vi "SubVI_Edge_Auto.vi"(8 "error in":errorcluster, 10 "Parameter_Edge":T3={"Parameter_Edge"={"ROI Descriptor"={"Global Rectangle"=[], "Contours"=[]}, "Edge Options"={"Edge Polarity"=0, "Kernel Size"=3, "Width"=3, "Minimum Edge Strength"=10.0, "Interpolation Type"=enum."Bilinear Fixed", "Data Processing Method"=enum."Average"}, "Scan Direction"=0, "Step Size"=5, "Auto"=FALSE}, "Group"="", "Color"=6618880, "Standard deviation"=0.0, "Pixel to Micrometer"=0.0, "Radius"=4} {"Parameter_Edge"."Edge Options"."Edge Polarity" items=["All Edges", "Rising Edges", "Falling Edges"]; "Parameter_Edge"."Edge Options"."Minimum Edge Strength" format="%.2f"; "Parameter_Edge"."Edge Options"."Width" step=2; "Parameter_Edge"."Edge Options"."Kernel Size" step=2; "Parameter_Edge"."Scan Direction" items=["Left To Right", "Right To Left", "Top To Bottom", "Bottom To Top"]; "Parameter_Edge"."ROI Descriptor"."Contours"."Type" items=["No Selection", "Point", "Line", "Rectangle", "Oval", "Polygon", "Free", "Annulus", "Unused2", "Unused3", "Broken Line", "Free Hand Line", "Rotated Rectangle"]}, 11 "Image in":T4) -> (0 "error out":errorcluster, 2 "Result_Edge":T5 {"MidPoint"."Y" format="%.2f"; "MidPoint"."X" format="%.2f"; "Line Segment"."Point 2"."Y" format="%.2f"; "Line Segment"."Point 2"."X" format="%.2f"; "Line Segment"."Point 1"."Y" format="%.2f"; "Line Segment"."Point 1"."X" format="%.2f"}, 3 "Image Out":T4)   [LabVIEW 2013]
uses:
  <vilib>/vision/Image Controls.llb/IMAQ Image.ctl
  <vilib>/vision/Measure.llb/Edge Options.ctl
  <vilib>/vision/Measure.llb/Edge Polarity.ctl
  <vilib>/vision/NI_Vision_Development_Module.lvlib
  <vilib>/Analysis/NI_AALBase.lvlib
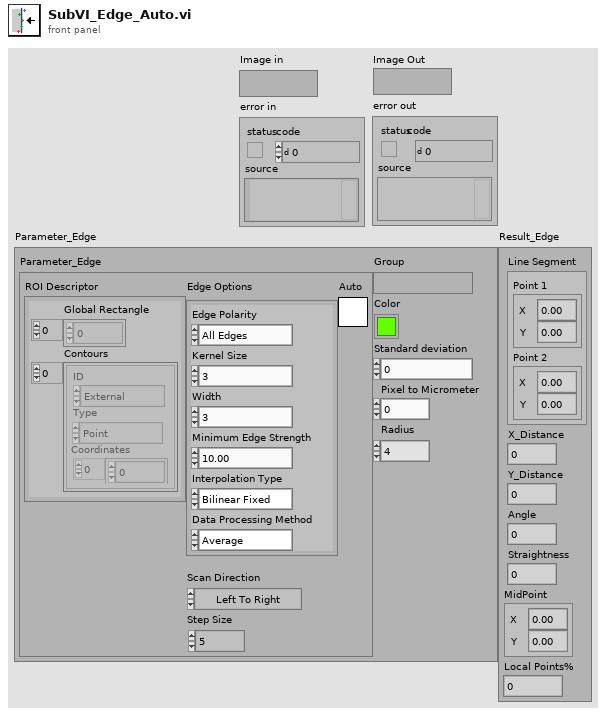
[diagram p1: front panel]
types:
  T1 = typedef "Edge Options.ctl" = cluster{"Edge Polarity":T2, "Kernel Size":u32, "Width":u32, "Minimum Edge Strength":sgl, "Interpolation Type":enum32{"Zero Order", "Bilinear", "Quadratic", "Cubic", "Bilinear Fixed"}, "Data Processing Method":enum32{"Average", "Median"}}
  T2 = typedef "Edge Polarity.ctl" = u32
  T3 = cluster{"Parameter_Edge":cluster{"ROI Descriptor":cluster{"Global Rectangle":i32[], "Contours":cluster{"ID":enum32{"External", "Internal"}, "Type":u32, "Coordinates":i32[]}[]}, "Edge Options":T1, "Scan Direction":u16, "Step Size":u32, "Auto":bool}, "Group":string, "Color":u32, "Standard deviation":dbl, "Pixel to Micrometer":dbl, "Radius":i32}
  T4 = typedef "IMAQ Image.ctl" = refnum<image>
  T5 = cluster{"Line Segment":cluster{"Point 1":cluster{"X":sgl, "Y":sgl}, "Point 2":cluster{"X":sgl, "Y":sgl}}, "X_Distance":dbl, "Y_Distance":dbl, "Angle":dbl, "Straightness":dbl, "MidPoint":cluster{"X":sgl, "Y":sgl}, "Local Points%":dbl}
  T6 = cluster{"ROI Descriptor":cluster{"Global Rectangle":i32[], "Contours":cluster{"ID":enum32{"External", "Internal"}, "Type":u32, "Coordinates":i32[]}[]}, "Edge Options":T1, "Scan Direction":u16, "Step Size":u32, "Auto":bool}
  T7 = cluster{"Point 1":cluster{"X":sgl, "Y":sgl}, "Point 2":cluster{"X":sgl, "Y":sgl}}
  T8 = cluster{"Point 1":cluster{"X":i32, "Y":i32}, "Point 2":cluster{"X":i32, "Y":i32}}
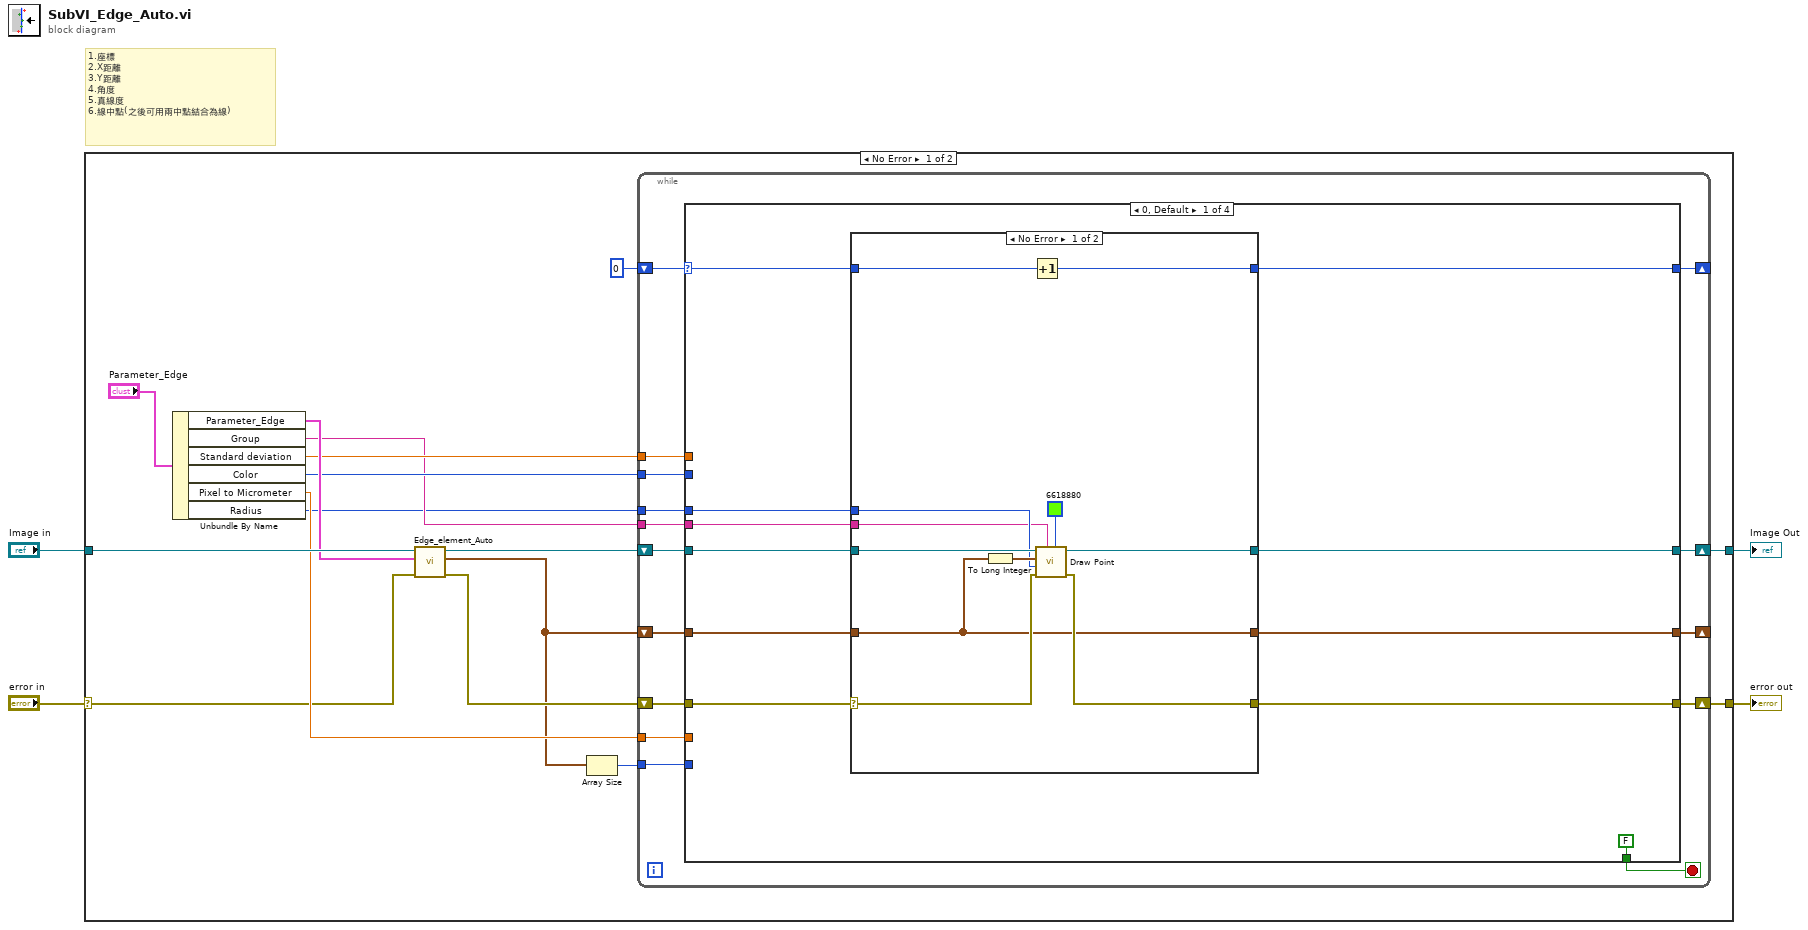
[diagram p0: block diagram]
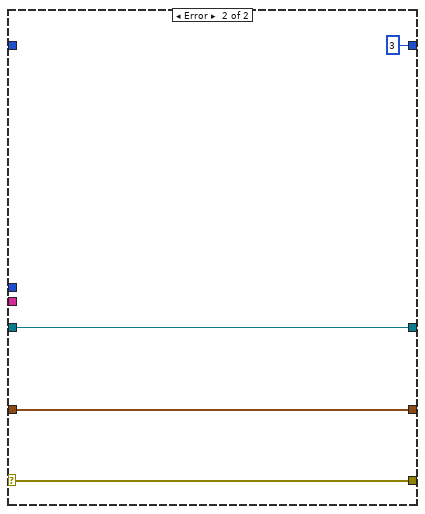
[diagram p2: hidden frame]
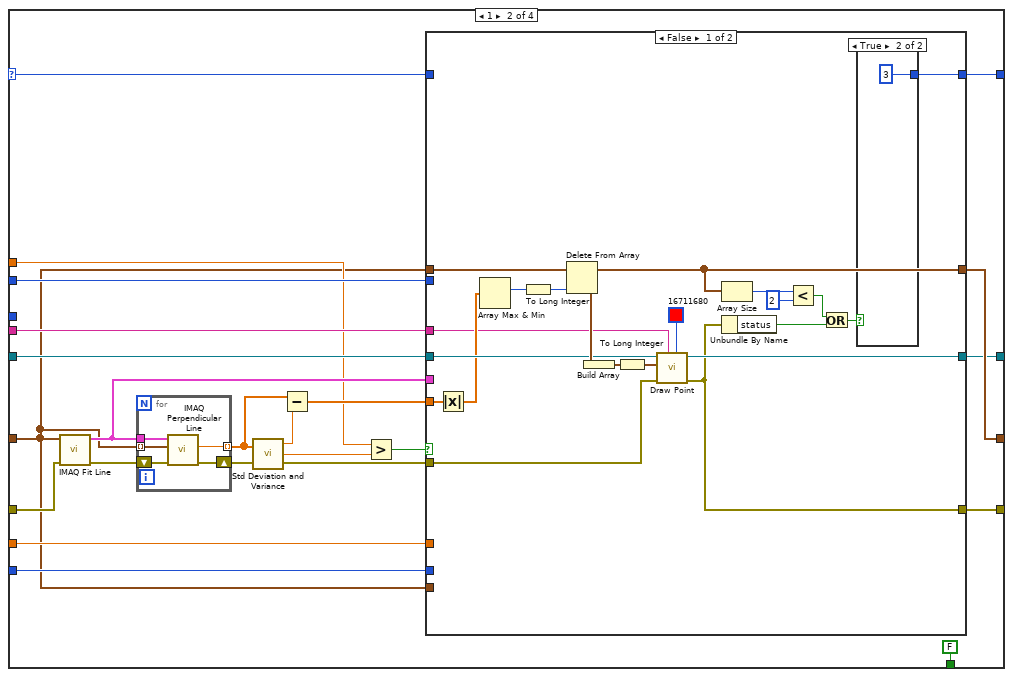
[diagram p3: hidden frame]
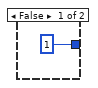
[diagram p4: hidden frame]
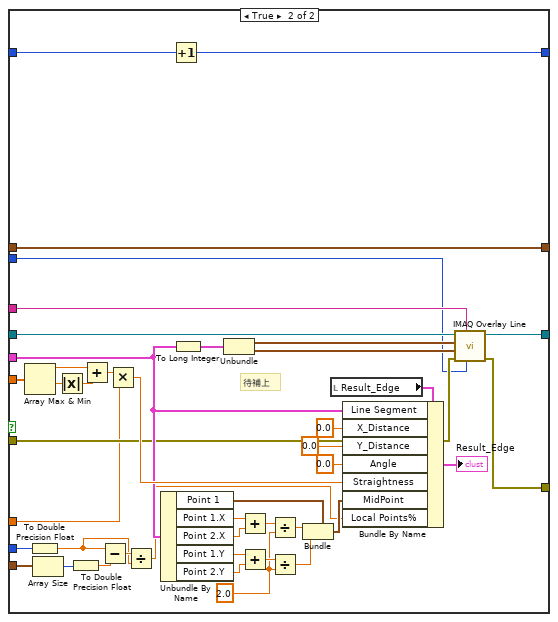
[diagram p5: hidden frame]
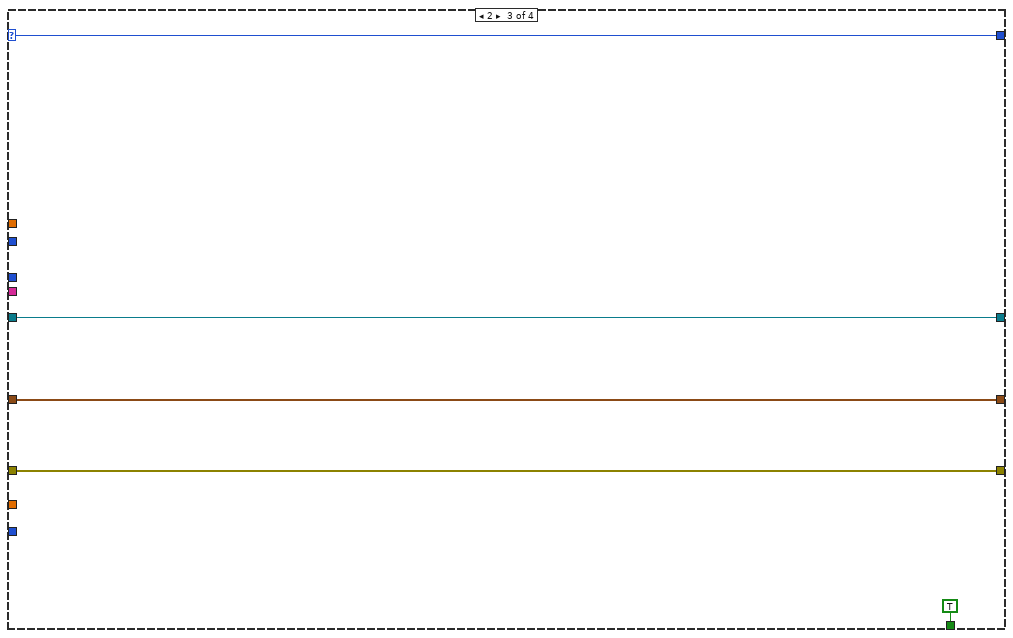
[diagram p6: hidden frame]
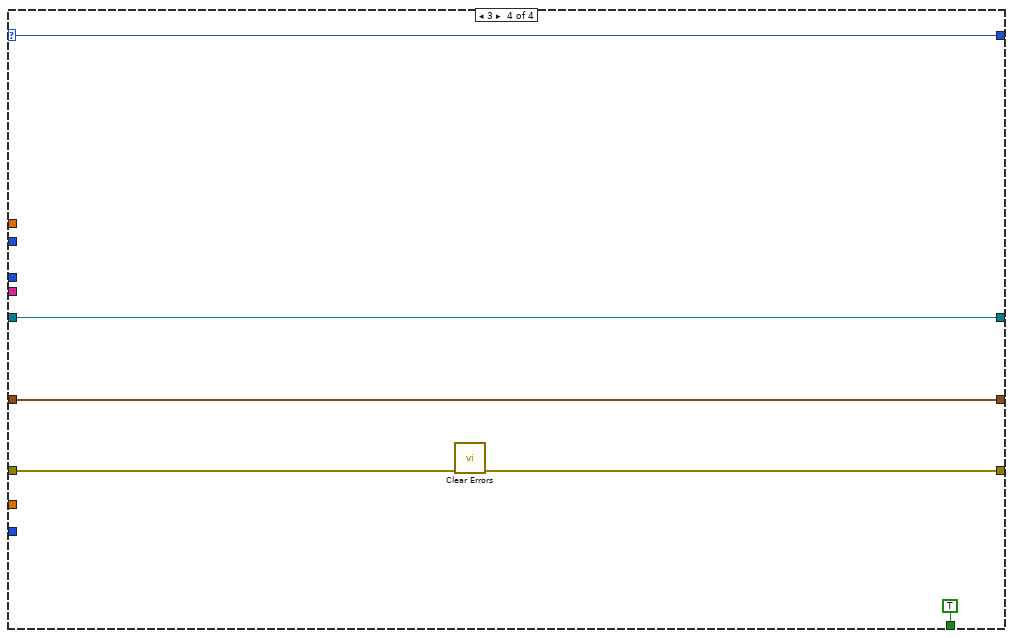
[diagram p7: hidden frame]
diagram:
  # "1.座標\n2.X距離\n3.Y距離\n4.角度\n5.真線度\n6.線中點(之後可用兩中點結合為線)"
  n1 = case shown="No Error" "error in" {
    selector: "error in" -> [w11 w167]
    tunnel: "Image in" -> [w18 w166]
    tunnel: [w10 w167] -> w2
    tunnel: [w9 w166] -> w1
    frame No Error {
      n2 = Unbundle By Name("Parameter_Edge") -> ("Parameter_Edge"=w15:T6, "Group"=w8:string, "Standard deviation"=w12:dbl, "Color"=w14:u32, "Pixel to Micrometer"=w13:dbl, "Radius"=w7:i32)
      n3 = call "Edge_element_Auto.vi"("Error In"=w11, "Parameter_Edge"=w15, "Image In"=w18) -> ("Error Out"=w19:errorcluster, "Location"=w6:cluster{"X":sgl, "Y":sgl}[], "Image Out"=w17:T4)  [unwired: 6 in]
      n4 = Array Size(array=w6) -> (size(s)=w5:i32)
      n5 = while {
        shift-right: [w33] -> _
        shift-left: 0 -> [w35]
        shift-right: [w32] -> w10
        shift-left: w19 -> [w34]
        shift-right: [w30] -> _
        shift-left: w6 -> [w31]
        shift-right: [w28] -> w9
        shift-left: w17 -> [w29]
        tunnel: w8 -> [w27]
        tunnel: w14 -> [w25]
        tunnel: w12 -> [w24]
        tunnel: w13 -> [w23]
        tunnel: w7 -> [w22]
        tunnel: w5 -> [w21]
        stop <- w26 stop-if-true
        n6 = case shown="0, Default" w35 {
          selector: w35 -> [w42 w70 w156 w160]
          tunnel: w34 -> [w40 w82 w159 w165]
          tunnel: [w41 w71 w156 w160] -> w33
          tunnel: [w44 w72 w159 w164] -> w32
          tunnel: [w38 w77 w157 w162] -> w30
          tunnel: w31 -> [w39 w62 w157 w162]
          tunnel: w29 -> [w46 w76 w158 w163]
          tunnel: [w45 w75 w158 w163] -> w28
          tunnel: w27 -> [w36 w74 _ _]
          tunnel: [FALSE FALSE TRUE TRUE] -> w26
          tunnel: w25 -> [_ w66 _ _]
          tunnel: w24 -> [_ w65 _ _]
          tunnel: w23 -> [_ w64 _ _]
          tunnel: w22 -> [w37 _ _ _]
          tunnel: w21 -> [_ w63 _ _]
          frame 0, Default {
            n7 = case shown="No Error" w40 {
              selector: w40 -> [w50 w59]
              tunnel: w46 -> [w56 w60]
              tunnel: [w55 w60] -> w45
              tunnel: [w53 w59] -> w44
              tunnel: w42 -> [w52 _]
              tunnel: [w51 3] -> w41
              tunnel: w39 -> [w49 w58]
              tunnel: [w49 w58] -> w38
              tunnel: w37 -> [w48 _]
              tunnel: w36 -> [w47 _]
              frame No Error {
                n8 = To Long Integer(number=w49) -> (32bit integer=w54:cluster{"X":i32, "Y":i32}[])
                n9 = Increment(x=w52) -> (x+1=w51:i32)
                n10 = call "Draw Point.vi"("Color"=u32 6618880 ("Circle radius"), "Group"=w47, "error in"=w50, "Radius"=w48, "Points"=w54, "Image In"=w56) -> ("error out"=w53:errorcluster, "Image Out"=w55:T4)  [unwired: 2 in]
              }
              frame Error {
              }
            }
          }
          frame 1 {
            n11 = call "IMAQ Fit Line"("error in (no error)"=w82, "Points"=w62) -> ("error out"=w81:errorcluster, "Line Segment"=w69:T7)  [unwired: 3 in, 5 out]
            n12 = for {
              tunnel: w69 -> [w154]
              tunnel: w62 -> [w153] mode=indexing
              tunnel: [w152] -> w79 mode=indexing
              shift-right: [w150] -> w73
              shift-left: w81 -> [w151]
              n13 = call "IMAQ Perpendicular Line"("error in (no error)"=w151, "Point"=w153, "Line"=w154) -> ("error out"=w150:errorcluster, "Distance"=w152:dbl)  [unwired: 6 in, 1 out]
            }
            n14 = call <vilib>:"Std Deviation and Variance.vi"("X"=w79) -> ("mean"=w80:dbl, "standard deviation"=w83:dbl)  [unwired: 1 in, 1 out]
            n15 = Subtract(x=w79, y=w80) -> (x-y=w68:dbl[])
            n16 = Greater?(x=w65, y=w83) -> (0:w78:bool)
            n17 = case shown="False" w78 {
              tunnel: w62 -> [w104 w147]
              tunnel: [w91 w147] -> w77
              tunnel: w76 -> [w98 w129]
              tunnel: [w97 w128] -> w75
              tunnel: w74 -> [w84 w127]
              tunnel: w73 -> [w95 w122]
              tunnel: [w93 w121] -> w72
              tunnel: [w94 w148] -> w71
              tunnel: w70 -> [_ w149]
              tunnel: w69 -> [_ w126]
              tunnel: w68 -> [w85 w146]
              tunnel: w66 -> [_ w116]
              tunnel: w64 -> [_ w115]
              tunnel: w63 -> [_ w112]
              tunnel: w62 -> [_ w114]
              frame False {
                n18 = Absolute Value(x=w85) -> (abs(x)=w86:dbl[])
                n19 = Array Max & Min(array=w86) -> (max index (indices)=w103:i32)  [unwired: 3 out]
                n20 = To Long Integer(number=w103) -> (32bit integer=w102:i32)
                n21 = Delete From Array(array=w104, index=w102) -> (deleted portion=w101:cluster{"X":sgl, "Y":sgl}, array with subset deleted=w91:cluster{"X":sgl, "Y":sgl}[])  [unwired: 1 in]
                n22 = Build Array(w101) -> (w99:cluster{"X":sgl, "Y":sgl}[])
                n23 = To Long Integer(number=w99) -> (32bit integer=w100:cluster{"X":i32, "Y":i32}[])
                n24 = call "Draw Point.vi"("Color"=u32 16711680 ("Circle radius"), "Group"=w84, "error in"=w95, "Points"=w100, "Image In"=w98) -> ("error out"=w93:errorcluster, "Image Out"=w97:T4)  [unwired: 3 in]
                n25 = Array Size(array=w91) -> (size(s)=w90:i32)
                n26 = Unbundle By Name(w93) -> ("status"=w92:bool)
                n27 = Less?(x=w90, y=2) -> (x < y?=w88:bool)
                n28 = Or(x=w88, y=w92) -> (x .or. y?=w87:bool)
                n29 = case shown="True" w87 {
                  tunnel: [1 3] -> w94
                  frame False {
                  }
                  frame True {
                  }
                }
              }
              frame True {
                w134 = sgl 2.0 ("y")
                # "待補上"
                n30 = Array Max & Min(array=w146) -> (max value=w143:dbl, min value=w144:dbl)  [unwired: 2 out]
                n31 = To Double Precision Float(number=w112) -> (double precision float=w109:dbl)
                n32 = Array Size(array=w114) -> (size(s)=w113:i32)
                n33 = Absolute Value(x=w144) -> (abs(x)=w145:dbl)
                n34 = To Double Precision Float(number=w113) -> (double precision float=w111:dbl)
                n35 = Add(x=w143, y=w145) -> (x+y=w142:dbl)
                n36 = Subtract(x=w109, y=w111) -> (x-y=w110:dbl)
                n37 = Multiply(x=w142, y=w115) -> (x*y=w141:dbl)
                n38 = Divide(x=w110, y=w109) -> (x/y=w107:dbl)
                n39 = Unbundle By Name(w126) -> ("Point 1"=w131:cluster{"X":sgl, "Y":sgl}, "Point 1.X"=w140:sgl, "Point 2.X"=w139:sgl, "Point 1.Y"=w137:sgl, "Point 2.Y"=w136:sgl)
                n40 = Increment(x=w149) -> (x+1=w148:i32)
                n41 = To Long Integer(number=w126) -> (32bit integer=w125:T8)
                n42 = Unbundle(w125) -> ("Point 1"=w124:cluster{"X":i32, "Y":i32}, "Point 2"=w123:cluster{"X":i32, "Y":i32})
                n43 = Add(x=w140, y=w139) -> (x+y=w138:sgl)
                n44 = Add(x=w137, y=w136) -> (x+y=w135:sgl)
                n45 = Divide(x=w138, y=w134) -> (x/y=w133:sgl)
                n46 = Divide(x=w135, y=w134) -> (x/y=w132:sgl)
                n47 = Bundle(cluster=w131, "X"=w133, "Y"=w132) -> (w130:cluster{"X":sgl, "Y":sgl})
                n48 = local read "Result_Edge"() -> (w108:T5)
                n49 = Bundle By Name(cluster=w108, "Line Segment"=w126, "X_Distance"=0.0, "Y_Distance"=0.0, "Angle"=0.0, "Straightness"=w141, "MidPoint"=w130, "Local Points%"=w107) -> (→"Result_Edge":T5)
                n50 = call "IMAQ Overlay Line"("Color"=w116, "Group"=w127, "error in (no error)"=w122, "End Point"=w123, "Start Point"=w124, "Image"=w129) -> ("error out"=w121:errorcluster, "Image Out"=w128:T4)  [unwired: 4 in]
              }
            }
          }
          frame 2 {
          }
          frame 3 {
            n51 = call <vilib>:"Clear Errors.vi"("error in (no error)"=w165) -> ("error out"=w164:errorcluster)  [unwired: 6 in]
          }
        }
      }
    }
    frame Error {
    }
  }
  "error out" <- w2
  "Image Out" <- w1
